vi "MoveHWP primitive.vi"(6 "tolerance":sgl, 7 "StopCtrl":bool, 8 "error in (no error)":errorcluster, 9 "DesiredAngle":sgl, 10 "HomeTheStage":bool, 11 "Automation Refnum in":refnum<k7>) -> (0 "error out":errorcluster, 1 "running error out":errorcluster, 2 "GetPosition_Position":sgl, 3 "GetStatusBits_Bits continual":i32 format="%b", 5 "CurrentAngle":sgl)   [LabVIEW 2013]
uses:
  <vilib>/Analysis/1siggen.llb/Ramp Pattern by Delta.vi
  <vilib>/Analysis/NI_AALBase.lvlib
panel:
  out "XY Graph":T1(graph)
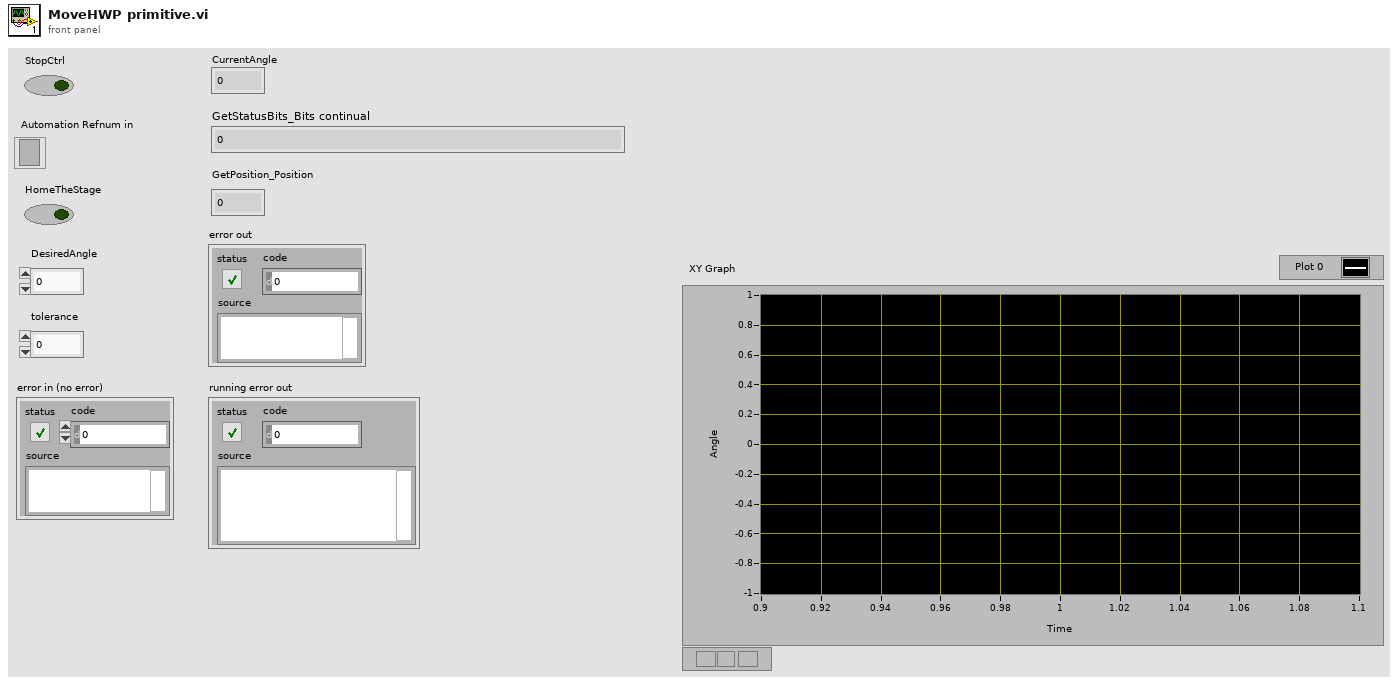
[diagram p1: front panel]
types:
  T1 = cluster{"Ramp Pattern":dbl[], "Array of Continuous Angles":dbl[]}
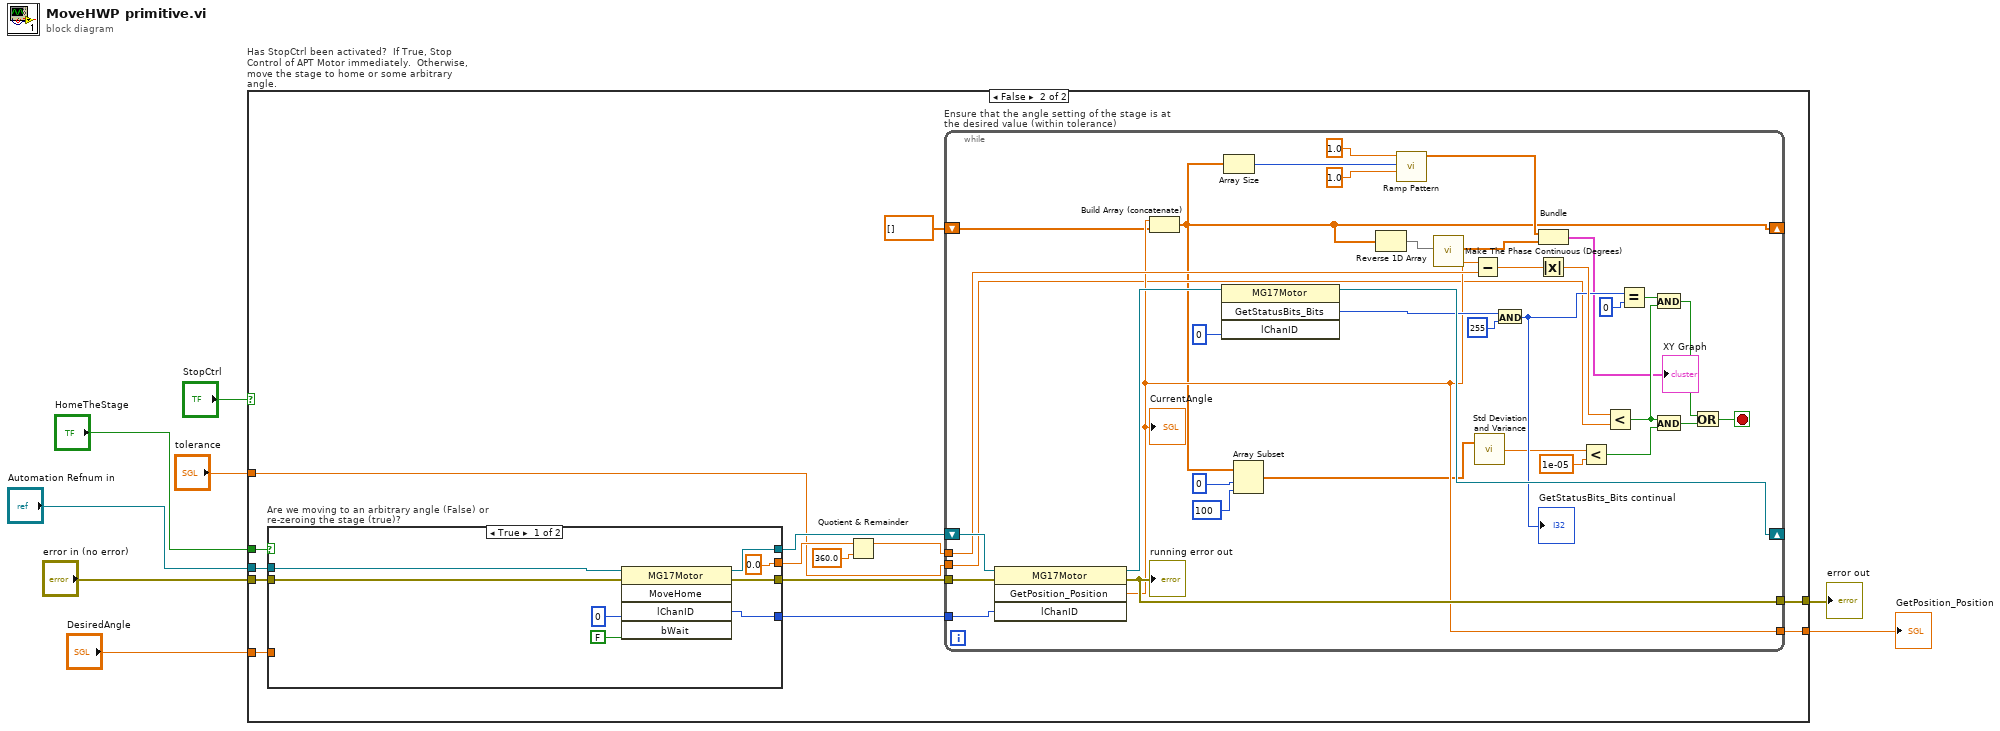
[diagram p0: block diagram]
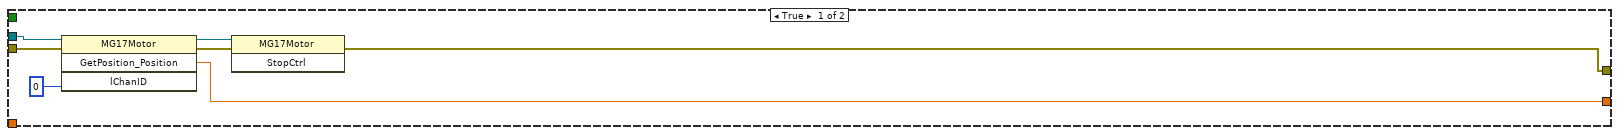
[diagram p2: hidden frame]
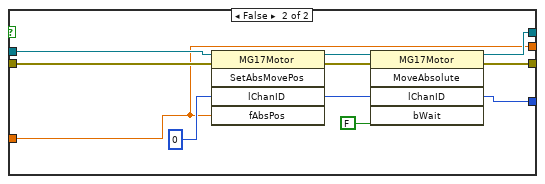
[diagram p3: hidden frame]
diagram:
  n1 = case "Has StopCtrl been activated?  If True, Stop Control of APT Motor immediately.  Otherwise, move the stage to home or some arbitrary angle." shown="False" "StopCtrl" {
    tunnel: "Automation Refnum in" -> [w15 w29]
    tunnel: "error in (no error)" -> [w14 w28]
    tunnel: [w10 w22] -> w3
    tunnel: [w9 w23] -> w2
    tunnel: "HomeTheStage" -> [_ w20]
    tunnel: "DesiredAngle" -> [_ w19]
    tunnel: "tolerance" -> [_ w18]
    frame True {
      n2 = invoke class="MG17Motor" method="GetPosition_Position"(reference=w15, error in=w14, "lChanID"=0) -> (reference out=w12:refnum<k7>, error out=w11:errorcluster, "GetPosition_Position"=w9:sgl)  [unwired: 1 in, 1 out]
      n3 = invoke class="MG17Motor" method="StopCtrl"(reference=w12, error in=w11) -> (error out=w10:errorcluster)  [unwired: 1 in, 2 out]
    }
    frame False {
      n4 = case "Are we moving to an arbitrary angle (False) or re-zeroing the stage (true)?" shown="True" w20 {
        tunnel: w29 -> [w71 w79]
        tunnel: w28 -> [w70 w78]
        tunnel: [w69 w77] -> w27
        tunnel: [sgl 0.0 ("Angle") w74] -> w26
        tunnel: [w67 w75] -> w25
        tunnel: [w66 w76] -> w24
        tunnel: w19 -> [_ w74]
        frame True {
          n5 = invoke class="MG17Motor" method="MoveHome"(reference=w71, error in=w70, "lChanID"=0, "bWait"=FALSE) -> (reference out=w69:refnum<k7>, error out=w66:errorcluster, "lChanID"=w67:i32)  [unwired: 1 in, 2 out]
        }
        frame False {
          n6 = invoke class="MG17Motor" method="SetAbsMovePos"(reference=w79, error in=w78, "lChanID"=0, "fAbsPos"=w74) -> (reference out=w84:refnum<k7>, error out=w83:errorcluster, "lChanID"=w82:i32)  [unwired: 1 in, 2 out]
          n7 = invoke class="MG17Motor" method="MoveAbsolute"(reference=w84, error in=w83, "lChanID"=w82, "bWait"=FALSE) -> (reference out=w77:refnum<k7>, error out=w76:errorcluster, "lChanID"=w75:i32)  [unwired: 1 in, 2 out]
        }
      }
      n8 = Quotient & Remainder(x=w26, y=sgl 360.0) -> (x-y*floor(x/y)=w17:sgl)  [unwired: 1 out]
      n9 = while "Ensure that the angle setting of the stage is at the desired value (within tolerance)" {
        tunnel: w25 -> [w65]
        tunnel: w24 -> [w63]
        tunnel: w17 -> [w62]
        tunnel: [w59] -> w22
        tunnel: [w50] -> w23
        shift-right: [w56] -> _
        shift-left: w27 -> [w64]
        shift-right: [w32] -> _
        shift-left: sgl[] [] -> [w49]
        tunnel: w18 -> [w40]
        stop <- w44 stop-if-true
        n10 = invoke class="MG17Motor" method="GetPosition_Position"(reference=w64, error in=w63, "lChanID"=w65) -> (reference out=w57:refnum<k7>, error out=w59:errorcluster, "GetPosition_Position"=w50:sgl)  [unwired: 1 in, 1 out]
        "running error out" <- w59
        "CurrentAngle" <- w50
        n11 = Build Array (concatenate)(w50, w49) -> (w32:sgl[])
        n12 = invoke class="MG17Motor" method="GetStatusBits_Bits"(reference=w57, "lChanID"=0) -> (reference out=w56:refnum<k7>, "GetStatusBits_Bits"=w55:i32)  [unwired: 2 in, 2 out]
        n13 = Array Size(array=w32) -> (size(s)=w35:i32)
        n14 = Array Subset(array=w32, index=0, length=100) -> (w46:sgl[])
        n15 = Reverse 1D Array(array=w32) -> (reversed array=w31:sgl[])
        n16 = call-poly <vilib>:"Ramp Pattern.vi"("start"=1.0, "end"=w35, "delta"=1.0) -> ("Ramp Pattern"=w34:dbl[])  [unwired: 6 in, 2 out]
        n17 = call "Make The Phase Continuous (Degrees).vi"("Array of Angles\nDiscontinuous"=w31) -> ("Array of Continuous Angles"=w30:dbl[])  [unwired: 10 in]
        n18 = Subtract(x=w50, y=w62) -> (x-y=w61:sgl)
        n19 = call <vilib>:"Std Deviation and Variance.vi"("X"=w46) -> ("standard deviation"=w45:dbl)  [unwired: 1 in, 2 out]
        n20 = And(x=w55, y=255) -> (x .and. y?=w53:i32)
        "GetStatusBits_Bits continual" <- w53
        n21 = Absolute Value(x=w61) -> (abs(x)=w60:sgl)
        n22 = Bundle("Ramp Pattern"=w34, "Array of Continuous Angles"=w30) -> (→"XY Graph":T1)  [unwired: 1 in]
        n23 = Less?(x=w45, y=1e-05) -> (x < y?=w42:bool)
        n24 = Less?(x=w60, y=w40) -> (x < y?=w38:bool)
        n25 = Equal?(x=w53, y=0) -> (x = y?=w51:bool)
        n26 = And(x=w51, y=w38) -> (x .and. y?=w43:bool)
        n27 = And(x=w38, y=w42) -> (x .and. y?=w39:bool)
        n28 = Or(x=w43, y=w39) -> (x .or. y?=w44:bool)
      }
    }
  }
  "error out" <- w3
  "GetPosition_Position" <- w2
